vi "Lesson 1-2 Compartmentalizing the acquisition.vi"() -> ()   [LabVIEW 2020]
uses:
  HRM-AQN-input_clust.ctl
panel:
  out "error out":errorcluster
  in  "stop":bool
  out "Waveform Chart":waveform(dbl)(graph)
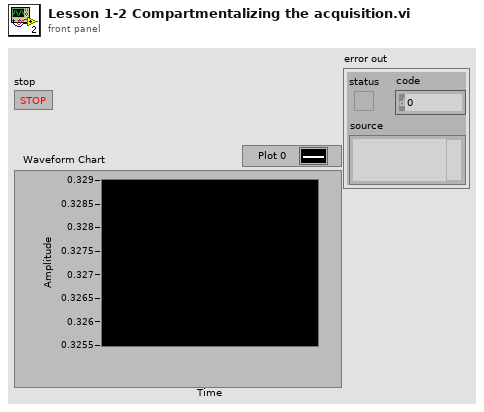
[diagram p1: front panel]
types:
  T1 = typedef "HRM-AQN-input_clust.ctl" = cluster{"physical channels":tag, "myDAQ task":refnum<k21>}
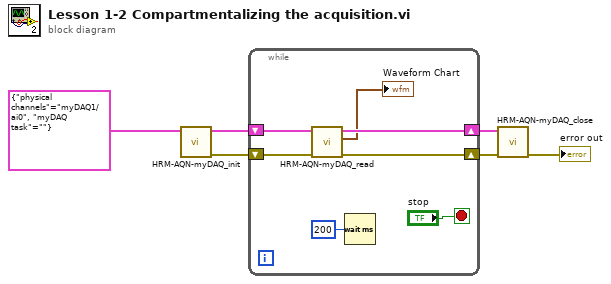
[diagram p0: block diagram]
diagram:
  n1 = call "HRM-AQN-myDAQ_init.vi"("AQN cluster in"=T1 {"physical channels"="myDAQ1/ai0", "myDAQ task"=""}) -> ("error out"=w6:errorcluster, "AQN cluster out"=w2:T1)  [unwired: 9 in]
  n2 = while {
    shift-right: [w8] -> w1
    shift-left: w2 -> [w9]
    shift-right: [w12] -> w5
    shift-left: w6 -> [w13]
    stop <- "stop" stop-if-true
    n3 = call "HRM-AQN-myDAQ_read.vi"("error in (no error)"=w13, "AQN cluster in"=w9) -> ("error out"=w12:errorcluster, "data"=→"Waveform Chart":waveform(dbl), "AQN cluster out"=w8:T1)  [unwired: 7 in]
    n4 = Wait (ms)(milliseconds to wait=u32 200) -> ()  [unwired: 1 out]
  }
  n5 = call "HRM-AQN-myDAQ_close.vi"("error in (no error)"=w5, "AQN cluster in"=w1) -> ("error out"=→"error out":errorcluster)  [unwired: 9 in]
